vi "GetNodeMenuOptions.vi"(0 "reference in":refnum<class "VINode.lvclass">, 1 "MousePos":T1 {"y" format="%.2f"; "x" format="%.2f"}, 5 "error in (no error)":errorcluster) -> (14 "reference out":refnum<class "VINode.lvclass">, 15 "MenuOptions":string[](array[string]), 19 "error out":errorcluster)   [LabVIEW 2016, in "VINode.lvclass"]
doc: "Gets the menu option"
uses:
  <resource>/Framework/Providers/Open_GDS/UML/VINode_class/VINode.lvclass
  C:/Program Files (x86)/National Instruments/LabVIEW 2016/resource/Framework/Providers/Open_GDS/UML/RectangularNode_class/RectangularNode.lvclass
  <resource>/Framework/Providers/Open_GDS/UML/General/Point/Point Point2D.ctl
  <resource>/Framework/Providers/Open_GDS/UML/RectangularNode_class/RectangularNode.lvclass
  <resource>/Framework/Providers/Open_GDS/UML/MultiLineString_class/MultiLineString.lvclass
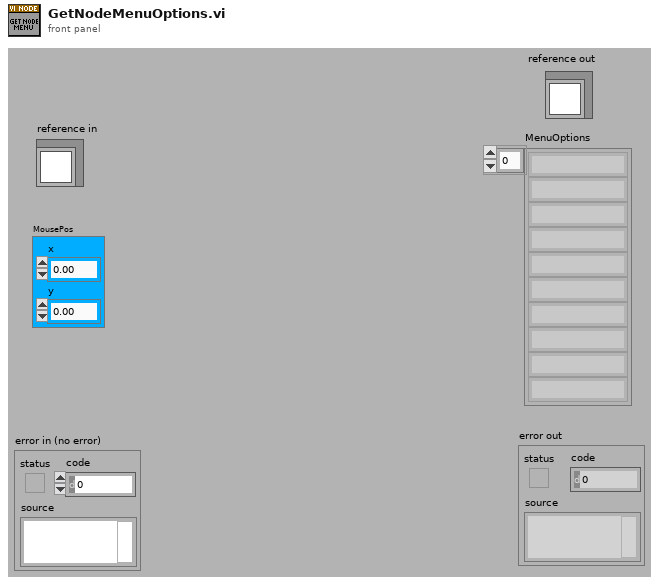
[diagram p1: front panel]
types:
  T1 = typedef "Point Point2D.ctl" = cluster{"x":dbl, "y":dbl}
  T2 = typedef "VINode.lvclass/ObjectAttributes.ctl" = cluster{"midHeight":dbl, "botHeight":dbl, "Name":refnum<class "MultiLineString.lvclass">, "DEFAULT_COMPARTMENT_HEIGHT":i32, "DEFAULT_WIDTH":i32, "DEFAULT_HEIGHT":i32, "VIPath":path, "Description":refnum<class "MultiLineString.lvclass">, "ShowDescription":bool}
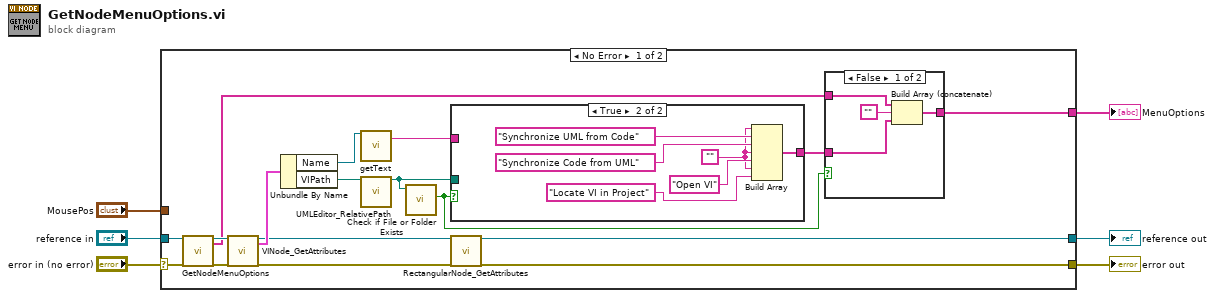
[diagram p0: block diagram]
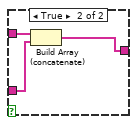
[diagram p3: hidden frame]
diagram:
  n1 = case shown="No Error" "error in (no error)" {
    selector: "error in (no error)" -> [w16 w37]
    tunnel: "reference in" -> [w17 w38]
    tunnel: [w11 w37] -> w5
    tunnel: [w10 w38] -> w4
    tunnel: [w9 _] -> w2
    tunnel: "MousePos" -> [_ _]
    frame No Error {
      n2 = call-parent "GetNodeMenuOptions.vi"("reference"=w17, "error in (no error)"=w16) -> ("reference out"=w19:refnum<class "VINode.lvclass">, "MenuOptions"=w18:string[], "error out"=w15:errorcluster)  [unwired: 15 in]
      n3 = call <resource>:"VINode_GetAttributes.vi"("reference in"=w19, "error in (no error)"=w15) -> ("reference out"=w13:refnum<class "VINode.lvclass">, "Data"=w14:T2, "error out"=w12:errorcluster)  [unwired: 1 in, 14 out]
      n4 = Unbundle By Name(w14) -> ("Name"=w22:refnum<class "MultiLineString.lvclass">, "VIPath"=w20:path)
      n5 = call-dynamic "getText.vi"("reference"=w22) -> ("text"=w21:string)  [unwired: 16 in, 2 out]
      n6 = call <resource>:"UMLEditor_RelativePath.vi"("Path In"=w20) -> ("ConvertToAbsolutePath(If possible)"=w8:path)  [unwired: 1 in, 17 out]
      n7 = call <vilib>:"Check if File or Folder Exists.vi"("path"=w8) -> ("file or folder exists?"=w7:bool)  [unwired: 8 in, 2 out]
      n8 = case shown="True" w7 {
        tunnel: [_ w29] -> w23
        tunnel: w21 -> [_ _]
        tunnel: w8 -> [_ _]
        frame False {
        }
        frame True {
          w25 = ""
          n9 = Build Array(w25, "Synchronize UML from Code" ("element"), "Synchronize Code from UML" ("element"), w25, "Open VI" ("element"), w25, "Locate VI in Project" ("element")) -> (w29:string[])
        }
      }
      n10 = call <resource>:"RectangularNode_GetAttributes.vi"("reference in"=w13, "error in (no error)"=w12) -> ("reference out"=w10:refnum<class "VINode.lvclass">, "error out"=w11:errorcluster)  [unwired: 14 in, 2 out]
      n11 = case shown="False" w7 {
        tunnel: [w33 w36] -> w9
        tunnel: w23 -> [w30 w35]
        tunnel: w18 -> [w32 w34]
        frame False {
          n12 = Build Array (concatenate)(w32, "", w30) -> (w33:string[])
        }
        frame True {
          n13 = Build Array (concatenate)(w34, w35) -> (w36:string[])
        }
      }
    }
    frame Error {
    }
  }
  "reference out" <- w4
  "error out" <- w5
  "MenuOptions" <- w2
